vi "2L20_IC_de_z_moy_sigma_dem.vi"(2 "z":dbl, 3 "S dem":dbl, 4 "m":dbl) -> (0 "Ic max":dbl, 1 "Ic min":dbl)   [LabVIEW 2010, in "lv_02.lvlib"]
doc: "IC ou RA à partir de la moyenne m, du quantile t de la loi de Gauss et de l'écart-type de la DEM"
uses:
  lv_02.lvlib
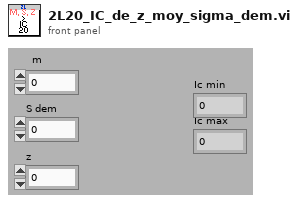
[diagram p1: front panel]
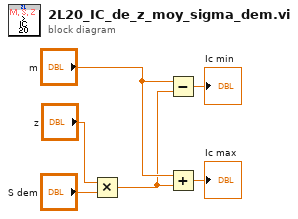
[diagram p0: block diagram]
diagram:
  n1 = Multiply(x="z", y="S dem") -> (x*y=w3:dbl)
  n2 = Subtract(x="m", y=w3) -> (x-y=→"Ic min":dbl)
  n3 = Add(x="m", y=w3) -> (x+y=→"Ic max":dbl)
